vi "GlobalArduinoNew.vi"() -> ()   [LabVIEW 2012]
uses:
  <vilib>/LabVIEW Interface for Arduino/Type Defs/Arduino Resource.ctl
  <vilib>/LabVIEW Interface for Arduino/Type Defs/Board Type.ctl
  <vilib>/LabVIEW Interface for Arduino/LabVIEW Interface for Arduino.lvlib
panel:
  out "arduino semaphore":T1
  out "valve pins":u8[](array[numeric])=[14, 16, 18, 17]
  in  "Last position command time":u64[](array[numeric])=[0, 0, 0, 4185119]
  out "servo pins":u8[](array[numeric])=[3, 5, 6, 9]
  out "error out":errorcluster={"status"=FALSE, "code"=1073676294, "source"="VISA Read in LabVIEW Interface for Arduino.lvlib:Send Receive.vi->LabVIEW Interface for Arduino.lvlib:Digital Read Pin.vi->readLightBarriersNew.vi->testNewArduino.vi"}
  out "Arduino Resource":T2={"VISA resource"="COM3", "Board Type"=enum."Uno", "Connection Type"=enum."USB / Serial", "Bytes Per Packet (15)"=15}
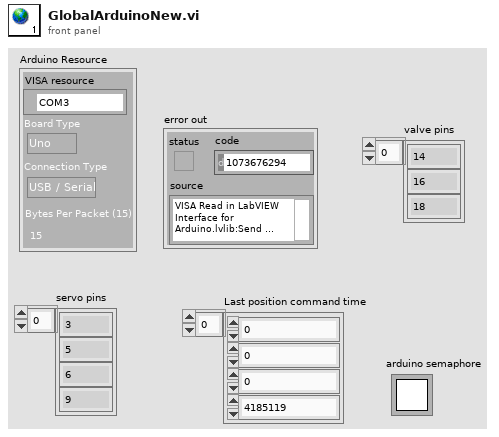
[diagram p1: front panel]
types:
  T1 = typedef "Semaphore RefNum" = refnum<k1>
  T2 = typedef "LabVIEW Interface for Arduino.lvlib/Arduino Resource.ctl" = cluster{"VISA resource":refnum<visa-resource-name>, "Board Type":T3, "Connection Type":enum8{"USB / Serial"}, "Bytes Per Packet (15)":u8}
  T3 = typedef "LabVIEW Interface for Arduino.lvlib/Board Type.ctl" = enum16{"Uno", "Dimuelanove w/Atmega 328", "Mega 2560"}
diagram:
